vi "color_detection.vi"() -> ()   [LabVIEW 2017]
uses:
  <vilib>/userdefined/High Color/IMAQdx.ctl
  <vilib>/vision/driver/NI_Vision_Acquisition_Software.lvlib
  <vilib>/vision/NI_Vision_Development_Module.lvlib
panel:
  out "rouge":bool
  out "bleu":bool
  out "vert":bool
  out "Color Spectrum":dbl[](array[numeric]) format="%.2f"
  in  "Color Sensitivity":u32(ring) items=["Low", "Medium", "High"]
  out "Image":T1(plugin-control)
  in  "stop":bool
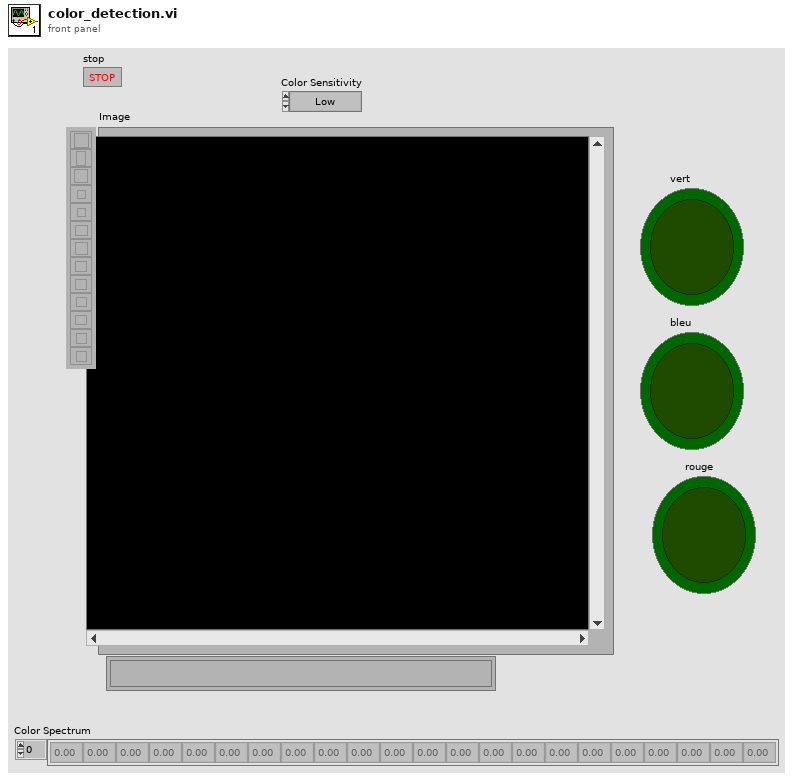
[diagram p1: front panel]
types:
  T1 = typedef "IMAQ Image.ctl" = refnum<image>
  T2 = typedef "IMAQdx.ctl" = refnum<k21>
  T3 = cluster{"Global Rectangle":i32[], "Contours":cluster{"Contour Type":u32, "ROI Type":u32, "Points":i32[]}[]}
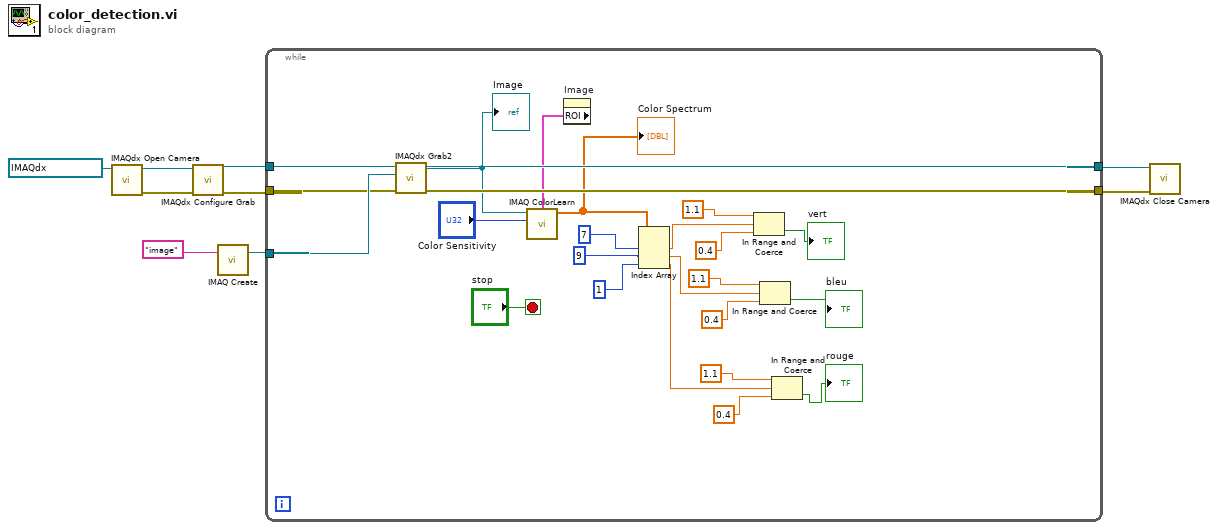
[diagram p0: block diagram]
diagram:
  n1 = call <vilib>:"IMAQdx Open Camera.vi"("Session In"=T2 "cam0") -> ("error out"=w8:errorcluster, "Session Out"=w9:T2)  [unwired: 9 in]
  n2 = call <vilib>:"IMAQdx Configure Grab.vi"("error in"=w8, "Session In"=w9) -> ("error out"=w4:errorcluster, "Session Out"=w5:T2)  [unwired: 8 in]
  n3 = call "IMAQ Create"("Image Name"="image") -> ("New Image"=w6:T1)  [unwired: 4 in, 1 out]
  n4 = while {
    tunnel: w6 -> [w34]
    tunnel: w5 -> [w33]
    tunnel: w4 -> [w32]
    tunnel: [w31] -> w3
    tunnel: [w30] -> w2
    stop <- "stop" stop-if-true
    n5 = call <vilib>:"IMAQdx Grab2.vi"("error in"=w32, "Image In"=w34, "Session In"=w33) -> ("error out"=w30:errorcluster, "Image Out"=w28:T1, "Session Out"=w31:T2)  [unwired: 5 in, 1 out]
    "Image" <- w28
    n6 = property on="Image" class="ImageControl"() -> ("ROI"=w26:T3)  [unwired: 2 in, 2 out]
    n7 = call "IMAQ ColorLearn"("ROI Descriptor"=w26, "Image"=w28, "Color Sensitivity"="Color Sensitivity") -> ("Color Spectrum"=w25:dbl[])  [unwired: 5 in, 1 out]
    "Color Spectrum" <- w25
    n8 = Index Array(array=w25, index #1=7 ("index"), index #2=9 ("index"), index #3=1 ("index")) -> (element #1=w22:dbl, element #2=w16:dbl, element #3=w11:dbl)
    n9 = In Range and Coerce(upper limit=1.1, x=w22, lower limit=0.4) -> (In Range?=→"vert":bool)  [unwired: 1 out]
    n10 = In Range and Coerce(upper limit=1.1, x=w16, lower limit=0.4) -> (In Range?=→"bleu":bool)  [unwired: 1 out]
    n11 = In Range and Coerce(upper limit=1.1, x=w11, lower limit=0.4) -> (In Range?=→"rouge":bool)  [unwired: 1 out]
  }
  n12 = call <vilib>:"IMAQdx Close Camera.vi"("error in"=w2, "Session In"=w3) -> ()  [unwired: 9 in, 1 out]
